vi "Get Feed ID.vi"(0 "SystemLink repo in":T1, 5 "feed name":string, 11 "error in (no error)":errorcluster) -> (4 "SystemLink repo out":T1, 6 "feed ID":string, 15 "error out":errorcluster)   [LabVIEW 2017, in "SystemLink_Repo_API.lvlib"]
doc: "Returns the Feed ID for the specified Feed Name.\n\nError Handling:\nReturns an error if the specified feed does not exist in the SystemLink repository."
uses:
  SystemLink_Repo_API.lvlib
  systemlink repo.ctl
  <vilib>/httpClient/ClientHandle.ctl
  <vilib>/httpClient/LabVIEWHTTPClient.lvlib
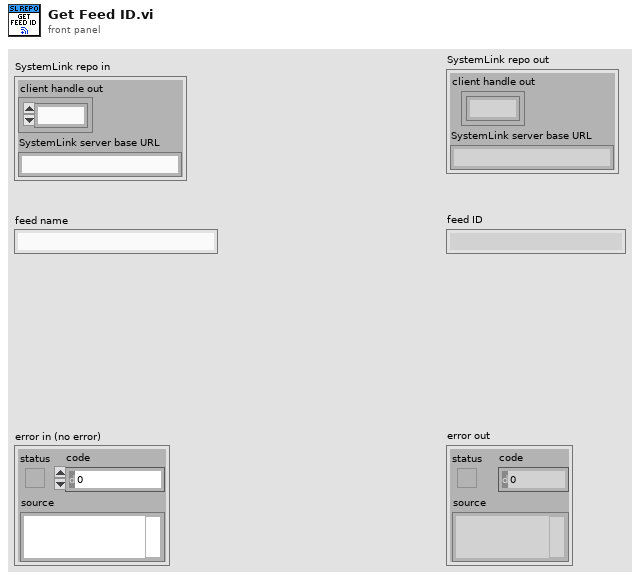
[diagram p1: front panel]
types:
  T1 = typedef "SystemLink_Repo_API.lvlib/systemlink repo.ctl" = cluster{"client handle out":T2, "SystemLink server base URL":string}
  T2 = typedef "LabVIEWHTTPClient.lvlib/ClientHandle.ctl" = refnum<k1>
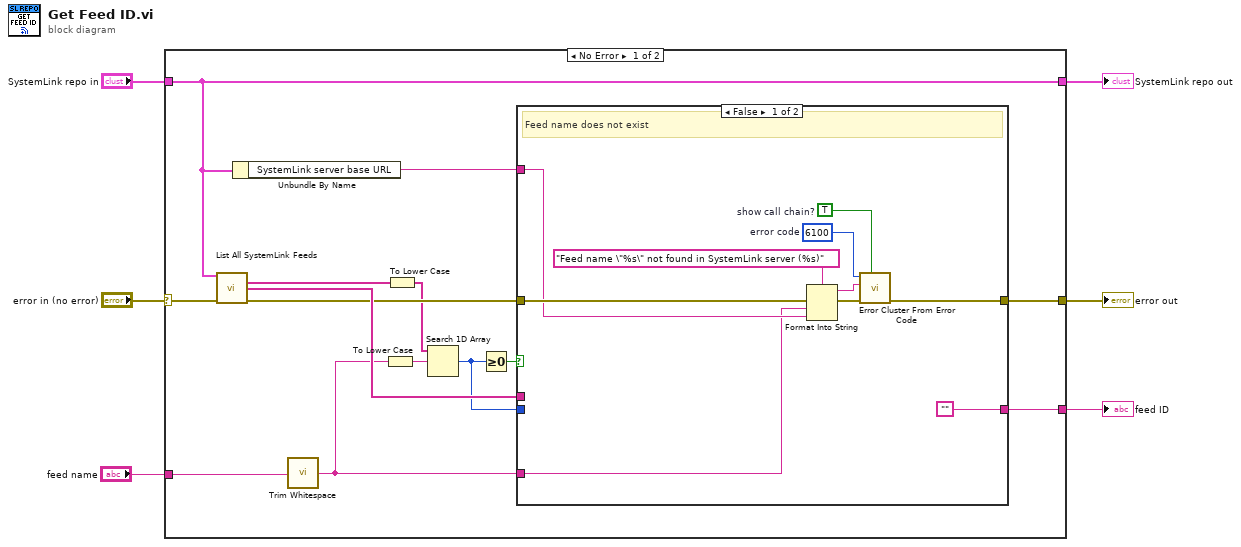
[diagram p0: block diagram]
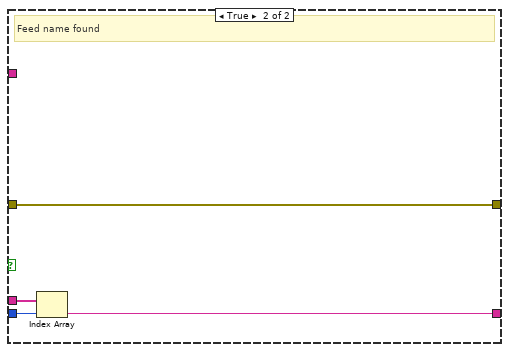
[diagram p2: hidden frame]
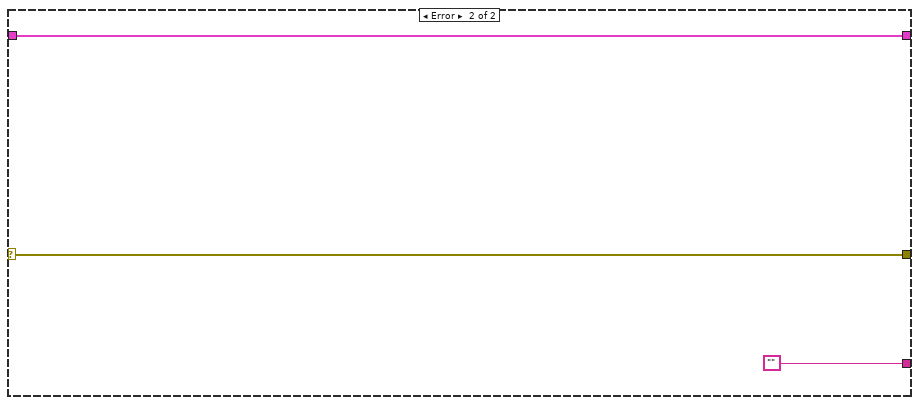
[diagram p3: hidden frame]
diagram:
  n1 = case shown="No Error" "error in (no error)" {
    selector: "error in (no error)" -> [w19 w37]
    tunnel: "SystemLink repo in" -> [w13 w36]
    tunnel: [w10 w37] -> w5
    tunnel: [w13 w36] -> w3
    tunnel: "feed name" -> [w20 _]
    tunnel: [w9 "" ("headers")] -> w1
    frame No Error {
      n2 = call "List All SystemLink Feeds.vi"("SystemLink repo in"=w13, "error in (no error)"=w19) -> ("SystemLink Feed Names"=w18:string[], "SystemLink Feed IDs"=w17:string[], "error out"=w14:errorcluster)  [unwired: 10 in, 1 out]
      n3 = Unbundle By Name(w13) -> ("SystemLink server base URL"=w12:string)
      n4 = call <vilib>:"Trim Whitespace.vi"("string"=w20) -> ("trimmed string"=w11:string)  [unwired: 1 in]
      n5 = To Lower Case(string=w11) -> (all lower case string=w8:string)
      n6 = To Lower Case(string=w18) -> (all lower case string=w7:string[])
      n7 = Search 1D Array(1D array=w7, element=w8) -> (index of element=w16:i32)  [unwired: 1 in]
      n8 = Greater Or Equal To 0?(x=w16) -> (x >= 0?=w15:bool)
      n9 = case shown="False" w15 {
        tunnel: w17 -> [_ w34]
        tunnel: w16 -> [_ w33]
        tunnel: w14 -> [w25 w31]
        tunnel: ["" w32] -> w9
        tunnel: [w22 w31] -> w10
        tunnel: w12 -> [w24 _]
        tunnel: w11 -> [w23 _]
        frame False {
          w26 = TRUE  # show call chain?
          w27 = 6100  # error code
          # "Feed name does not exist"
          n10 = Format Into String(format string="Feed name \"%s\" not found in SystemLink server (%s)", error in=w25, w23, w24) -> (resulting string=w28:string, error out=w30:errorcluster)  [unwired: 1 in]
          n11 = call <vilib>:"Error Cluster From Error Code.vi"("show call chain? (False)"=w26, "error in (no error)"=w30, "error message (\"\")"=w28, "error code (0)"=w27) -> ("error out"=w22:errorcluster)  [unwired: 5 in]
        }
        frame True {
          # "Feed name found"
          n12 = Index Array(array=w34, index=w33) -> (element=w32:string)
        }
      }
    }
    frame Error {
    }
  }
  "error out" <- w5
  "SystemLink repo out" <- w3
  "feed ID" <- w1
